vi "ConvertToFahrenheit.vi"(1 "Celcius":dbl) -> (0 "fahrenheit":dbl)   [LabVIEW 2021]
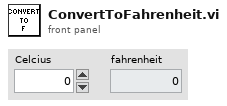
[diagram p1: front panel]
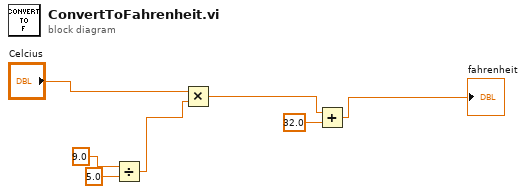
[diagram p0: block diagram]
diagram:
  n1 = Divide(x=9.0, y=5.0) -> (x/y=w5:dbl)
  n2 = Multiply(x="Celcius", y=w5) -> (x*y=w3:dbl)
  n3 = Add(x=w3, y=32.0) -> (x+y=→"fahrenheit":dbl)
